vi "Builder Status.Set Build Durations.vi"(10 "Build Durations":refnum<class "Memory.Pointer.U32.lvclass">, 11 "Builder Status in":refnum<class "Builder Status.lvclass">) -> (3 "Builder Status out":refnum<class "Builder Status.lvclass">)   [LabVIEW 2016, in "DSF.Engine.lvlib" / "Builder Status.lvclass"]
uses:
  Builder Status.lvclass
  Submodules/Memory/Source/Classes/Standard Types/Memory.Pointer.U32.lvclass
  Builder Status.lvclass/Builder Status.ctl
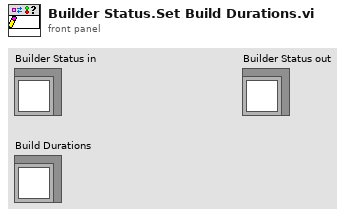
[diagram p1: front panel]
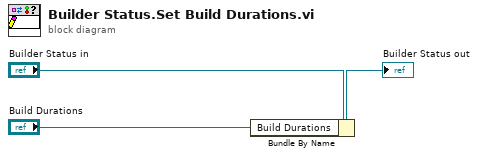
[diagram p0: block diagram]
diagram:
  n1 = Bundle By Name(cluster="Builder Status in", "Build Durations"="Build Durations") -> (→"Builder Status out":refnum<class "Builder Status.lvclass">)
